vi "BeamAnalyzer.vi"() -> ()   [LabVIEW 2011]
uses:
  <vilib>/Utility/miscctls.llb/LVCursorListTypeDef.ctl
  <vilib>/gmath/NI_Gmath.lvlib
panel:
  out "Numeric system matrix":dbl[][][](array[numeric])=[[[1.0, 0.0, 0.0, 0.0], [0.0, 1.0, 0.0, 0.0], [0.0, 0.0, 1.0, 0.0], [0.0, 0.0, 0.0, 1.0]], [[1.0, 80.487805, 0.0, 0.0], [-0.03333333333333333, -1.6829268333333331, 0.0, 0.0], [0.0, 0.0, 1.0, 80.487805], [0.0, 0.0, -0.03333333333333333, -1.6829268333333331]]]
  in  "Plot system fast":bool
  out "error":i32
  in  "number of points":u32=100
  out "Y array":dbl[][][](array[numeric])=[[[0.016448811606198852, 0.029859124074476537, 0.05248408284624274, 0.07654801361501866, 0.10102784566185909, 0.12568078844527222, 0.15042175156489726, 0.17521345233159344, 0.2000370270388385, 0.22488192072640245, 0.24974177088971808, 0.27461251566370104, 0.29949144088878066, 0.3243766643064927, 0.34926683968286143, 0.37416097876713134, 0.3990583397654776, 0.42395835504829776, 0.448860582885839, 0.47376467438639763, 0.49867035033051754, 0.5235773846104799, 0.5484855921779689, 0.5733948201305636, 0.5983049410232071, 0.6232158477826785, 0.6481274497941432, 0.6730396698563271, 0.6979524417884401, 0.7228657085317128, 0.7477794206302699, 0.7726935350057659, 0.797608013961588, 0.8225228243679736, 0.847437936990825, 0.8723533259355064, 0.8972689681832823, 0.9221848432028807, 0.9471009326233549, 0.9720172199572462, 0.9969336903652497, 1.0218503304553048, 1.0467671281103703, 1.0716840723402246, 1.0966011531534607, 1.121518361446548, 1.146435688907353, 1.1713531279309763, 1.1962706715461031, 1.2211883133503711, 1.246106047453491, 1.2710238684270556, 1.2959417712601402, 1.3208597513199272, 1.3457778043167032, 1.3706959262726768, 1.395614113494133, 1.4205323625465187, 1.4454506702321086, 1.470369033569936, 1.4952874497777342, 1.5202059162556534, 1.5451244305715506, 1.5700429904476831, 1.5949615937486477, 1.619880238470433, 1.644798922730467, 1.6697176447585562, 1.6946364028886234, 1.7195551955511643, 1.7444740212663505, 1.769392878637714, 1.7943117663463615, 1.8192306831456588, 1.844149627856351, 1.8690685993620708, 1.893987596605201, 1.918906618583061, 1.9438256643443839, 1.9687447329860648, 1.9936638236501494, 2.018582935521049, 2.043502067822955, 2.0684212198174454, 2.0933403908012576, 2.1182595801042217, 2.143178787087335, 2.168098011140974, 2.1930172516832216, 2.217936508158313, 2.242855780035183, 2.267775066806107, 2.2926943679854364, 2.317613683108406, 2.342533011730029, 2.3674523534240524, 2.3923717077819844, 2.417291074412175, 2.442210452938962, 2.4671298430018562], [0.016448811606198852, 0.029859124074476537, 0.05248408284624274, 0.07654801361501866, 0.10102784566185909, 0.12568078844527222, 0.15042175156489726, 0.17521345233159344, 0.2000370270388385, 0.22488192072640245, 0.24974177088971808, 0.27461251566370104, 0.29949144088878066, 0.3243766643064927, 0.34926683968286143, 0.37416097876713134, 0.3990583397654776, 0.42395835504829776, 0.448860582885839, 0.47376467438639763, 0.49867035033051754, 0.5235773846104799, 0.5484855921779689, 0.5733948201305636, 0.5983049410232071, 0.6232158477826785, 0.6481274497941432, 0.6730396698563271, 0.6979524417884401, 0.7228657085317128, 0.7477794206302699, 0.7726935350057659, 0.797608013961588, 0.8225228243679736, 0.847437936990825, 0.8723533259355064, 0.8972689681832823, 0.9221848432028807, 0.9471009326233549, 0.9720172199572462, 0.9969336903652497, 1.0218503304553048, 1.0467671281103703, 1.0716840723402246, 1.0966011531534607, 1.121518361446548, 1.146435688907353, 1.1713531279309763, 1.1962706715461031, 1.2211883133503711, 1.246106047453491, 1.2710238684270556, 1.2959417712601402, 1.3208597513199272, 1.3457778043167032, 1.3706959262726768, 1.395614113494133, 1.4205323625465187, 1.4454506702321086, 1.470369033569936, 1.4952874497777342, 1.5202059162556534, 1.5451244305715506, 1.5700429904476831, 1.5949615937486477, 1.619880238470433, 1.644798922730467, 1.6697176447585562, 1.6946364028886234, 1.7195551955511643, 1.7444740212663505, 1.769392878637714, 1.7943117663463615, 1.8192306831456588, 1.844149627856351, 1.8690685993620708, 1.893987596605201, 1.918906618583061, 1.9438256643443839, 1.9687447329860648, 1.9936638236501494, 2.018582935521049, 2.043502067822955, 2.0684212198174454, 2.0933403908012576, 2.1182595801042217, 2.143178787087335, 2.168098011140974, 2.1930172516832216, 2.217936508158313, 2.242855780035183, 2.267775066806107, 2.2926943679854364, 2.317613683108406, 2.342533011730029, 2.3674523534240524, 2.3923717077819844, 2.417291074412175, 2.442210452938962, 2.4671298430018562]]]
  out "X":dbl[][](array[numeric])=[[0.0, 1.515, 3.03, 4.545, 6.06, 7.574999999999999, 9.09, 10.604999999999999, 12.12, 13.635, 15.149999999999999, 16.665, 18.18, 19.695, 21.209999999999997, 22.724999999999998, 24.24, 25.755, 27.27, 28.784999999999997, 30.299999999999997, 31.814999999999998, 33.33, 34.845, 36.36, 37.875, 39.39, 40.904999999999994, 42.419999999999995, 43.934999999999995, 45.449999999999996, 46.964999999999996, 48.48, 49.995, 51.51, 53.025, 54.54, 56.055, 57.56999999999999, 59.084999999999994, 60.599999999999994, 62.114999999999995, 63.629999999999995, 65.145, 66.66, 68.175, 69.69, 71.205, 72.72, 74.235, 75.75, 77.265, 78.78, 80.295, 81.80999999999999, 83.32499999999999, 84.83999999999999, 86.35499999999999, 87.86999999999999, 89.38499999999999, 90.89999999999999, 92.41499999999999, 93.92999999999999, 95.445, 96.96, 98.475, 99.99, 101.505, 103.02, 104.535, 106.05, 107.565, 109.08, 110.595, 112.11, 113.62499999999999, 115.13999999999999, 116.65499999999999, 118.16999999999999, 119.68499999999999, 121.19999999999999, 122.71499999999999, 124.22999999999999, 125.74499999999999, 127.25999999999999, 128.775, 130.29, 131.80499999999998, 133.32, 134.83499999999998, 136.35, 137.86499999999998, 139.38, 140.89499999999998, 142.41, 143.92499999999998, 145.44, 146.95499999999998, 148.47, 149.98499999999999]]
  in  "Wavelength":dbl=0.00085
  out "q out":T1(array[cluster])=[{"qx"={"Re"="((z)*((1)+(0)*(0))+(1)*((1)*(0)+(0)*((1)^2 +(0)^2)))/((1)^2 + 2*(0)*(1)*(0)+(0)^2 *((1)^2 + (0)^2))", "Im"="(-(z)*(0)*(1)+(1)*(1)*(1))/((1)^2 + 2*(0)*(1)*(0)+(0)^2 *((1)^2 +(0)^2))"}, "qy"={"Re"="((z)*((1)+(0)*(0))+(1)*((1)*(0)+(0)*((1)^2 +(0)^2)))/((1)^2 + 2*(0)*(1)*(0)+(0)^2 *((1)^2 + (0)^2))", "Im"="(-(z)*(0)*(1)+(1)*(1)*(1))/((1)^2 + 2*(0)*(1)*(0)+(0)^2 *((1)^2 +(0)^2))"}}]
  in  "q in":T2={"qx"={"Re"="0", "Im"="1"}, "qy"={"Re"="0", "Im"="1"}}
  in  "Parameters":cluster{"Name":string, "Value":string}[](array[cluster])=[{"Name"="d0", "Value"="0"}, {"Name"="z", "Value"="x"}, {"Name"="f1", "Value"="30"}, {"Name"="d1", "Value"="80.487805"}]
  out "System plot":cluster{dbl[], dbl[]}[](graph)
  in  "Plot system":bool
  in  "LensHeight":u32=20
  out "Axis vertical pos":i16=63
  in  "Horizontal initial pos":dbl
  out "Horizontal pixels":u32=898
  in  "Horizontal final point":dbl=200.0
  in  "System matrix":string[][][](array[string])=[[["1", "z", "0", "0"], ["0", "1", "0", "0"], ["0", "0", "1", "z"], ["0", "0", "0", "1"]]]
  in  "Compute System":bool
  in  "Element cluster":T3
  in  "Element array":T4(array[cluster])=[{"Element type"="Spherical lens", "Position"="80.487805", "Parameters"=[{"Name"="f1", "Value"="30"}, {"Name"="d1", "Value"="80.487805"}]}]
  in  "Stop":bool
  in  "Objects":T5(tab)
  in  "Lens type":T6(radio)
  in  "Position":string="150"
  in  "Focal length":string="100"
  in  "Add lens":bool
  out "System plot":picture
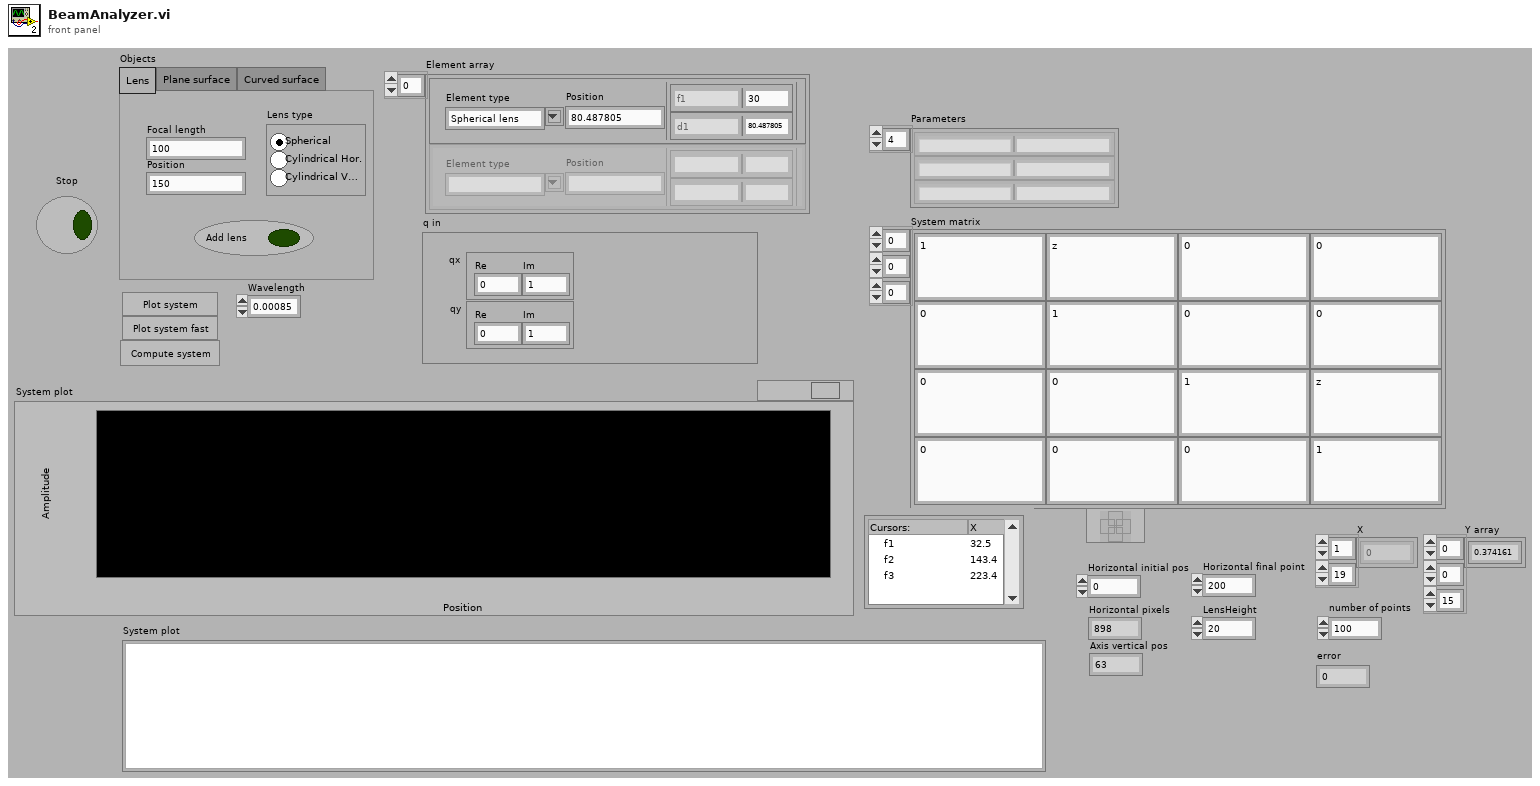
[diagram p1: front panel]
types:
  T1 = cluster{"qx":cluster{"Re":string, "Im":string}, "qy":cluster{"Re":string, "Im":string}}[]
  T2 = cluster{"qx":cluster{"Re":string, "Im":string}, "qy":cluster{"Re":string, "Im":string}}
  T3 = cluster{"Element type":string, "Position":string, "Parameters":cluster{"Name":string, "Value":string}[]}
  T4 = cluster{"Element type":string, "Position":string, "Parameters":cluster{"Name":string, "Value":string}[]}[]
  T5 = enum32{"Lens", "Plane surface", "Curved surface"}
  T6 = enum32{"Spherical", "Cylindrical Hor.", "Cylindrical Vert."}
  T7 = typedef "LVCursorListTypeDef.ctl" = cluster{"Name":string, "Color":u32, "Style":u8, "Point Style":u8, "Name Visible":bool, "Allow Drag":bool, "Cursor Mode":u32, "Plot":i32, "Index":i32, "Position":cluster{"X":dbl, "Y":dbl}, "X Scale":u32, "Y Scale":u32, "Watch Plots":i32[], "Watch All Plots":bool, "Plot Area":i32, "Label Offset":cluster{"X":dbl, "Y":dbl}}[]
  T8 = cluster{"Name":string, "Color":u32, "Style":u8, "Point Style":u8, "Name Visible":bool, "Allow Drag":bool, "Cursor Mode":u32, "Plot":i32, "Index":i32, "Position":cluster{"X":dbl, "Y":dbl}, "X Scale":u32, "Y Scale":u32, "Watch Plots":i32[], "Watch All Plots":bool, "Plot Area":i32, "Label Offset":cluster{"X":dbl, "Y":dbl}}
  T9 = typedef "LVBoundsTypeDef.ctl" = cluster{"Width":u32, "Height":u32}
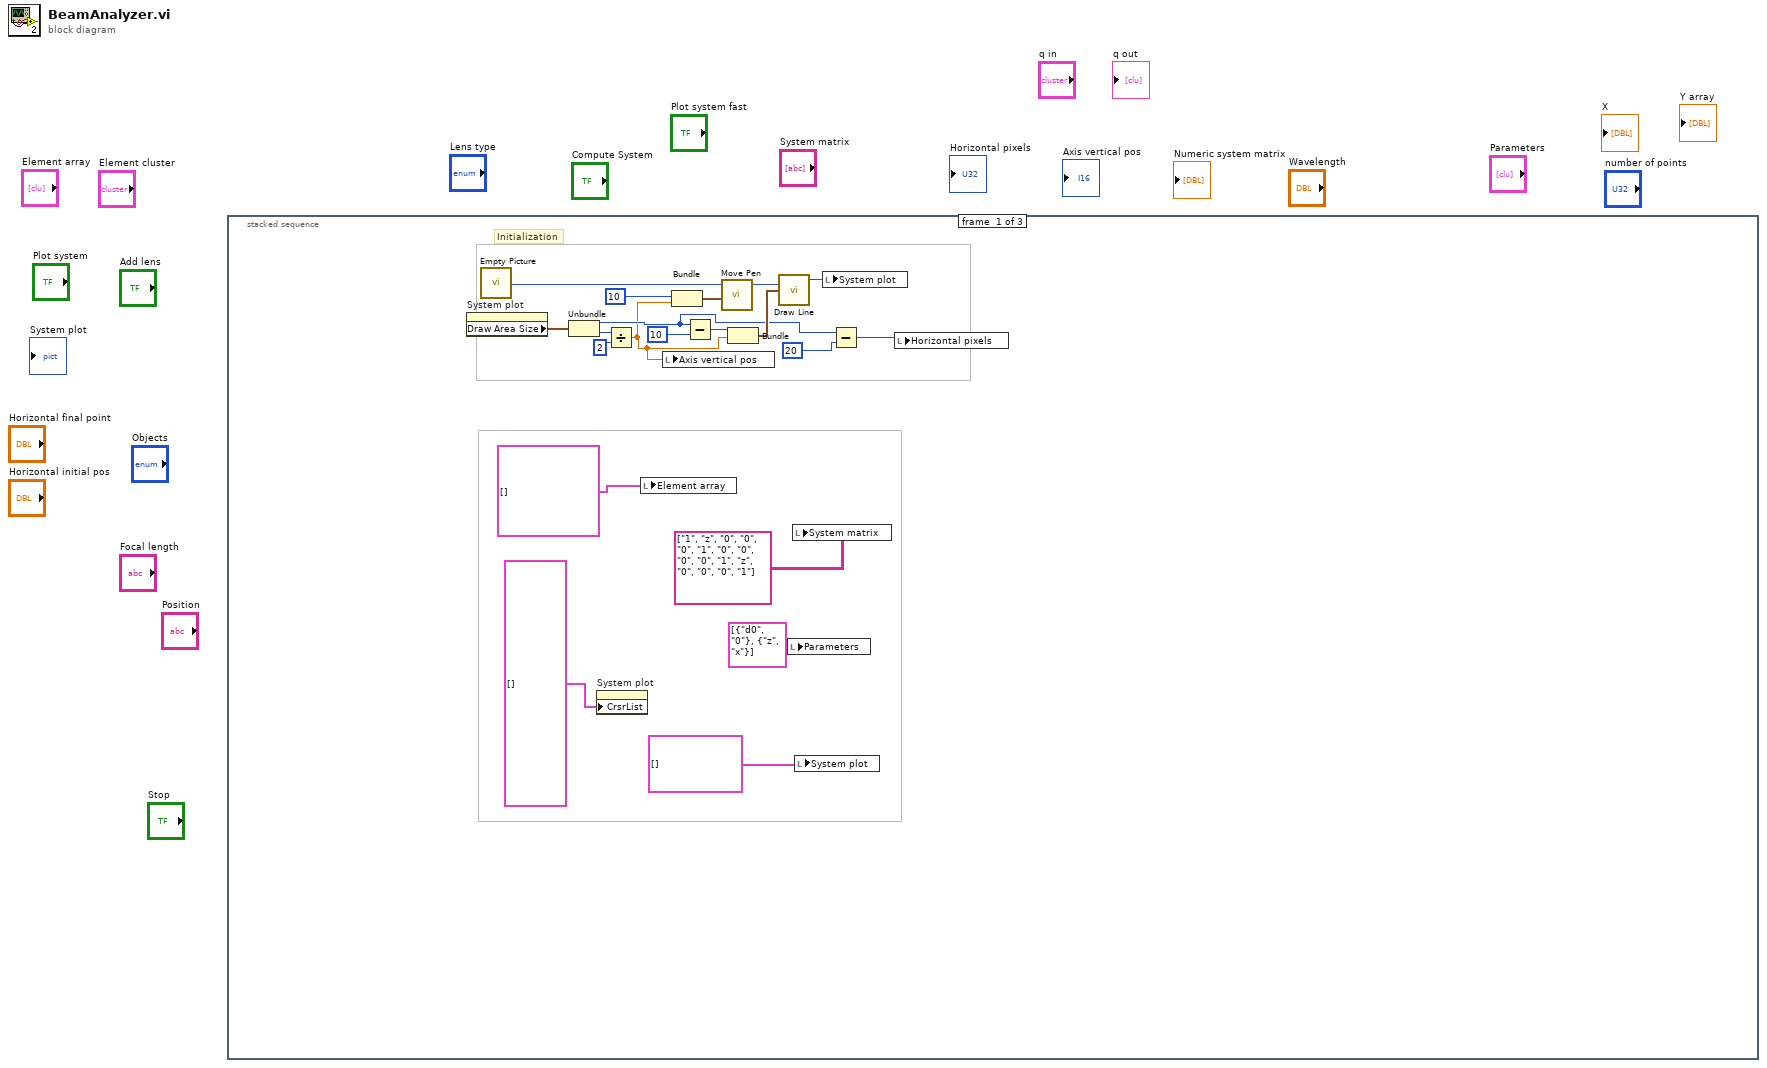
[diagram p0: block diagram]
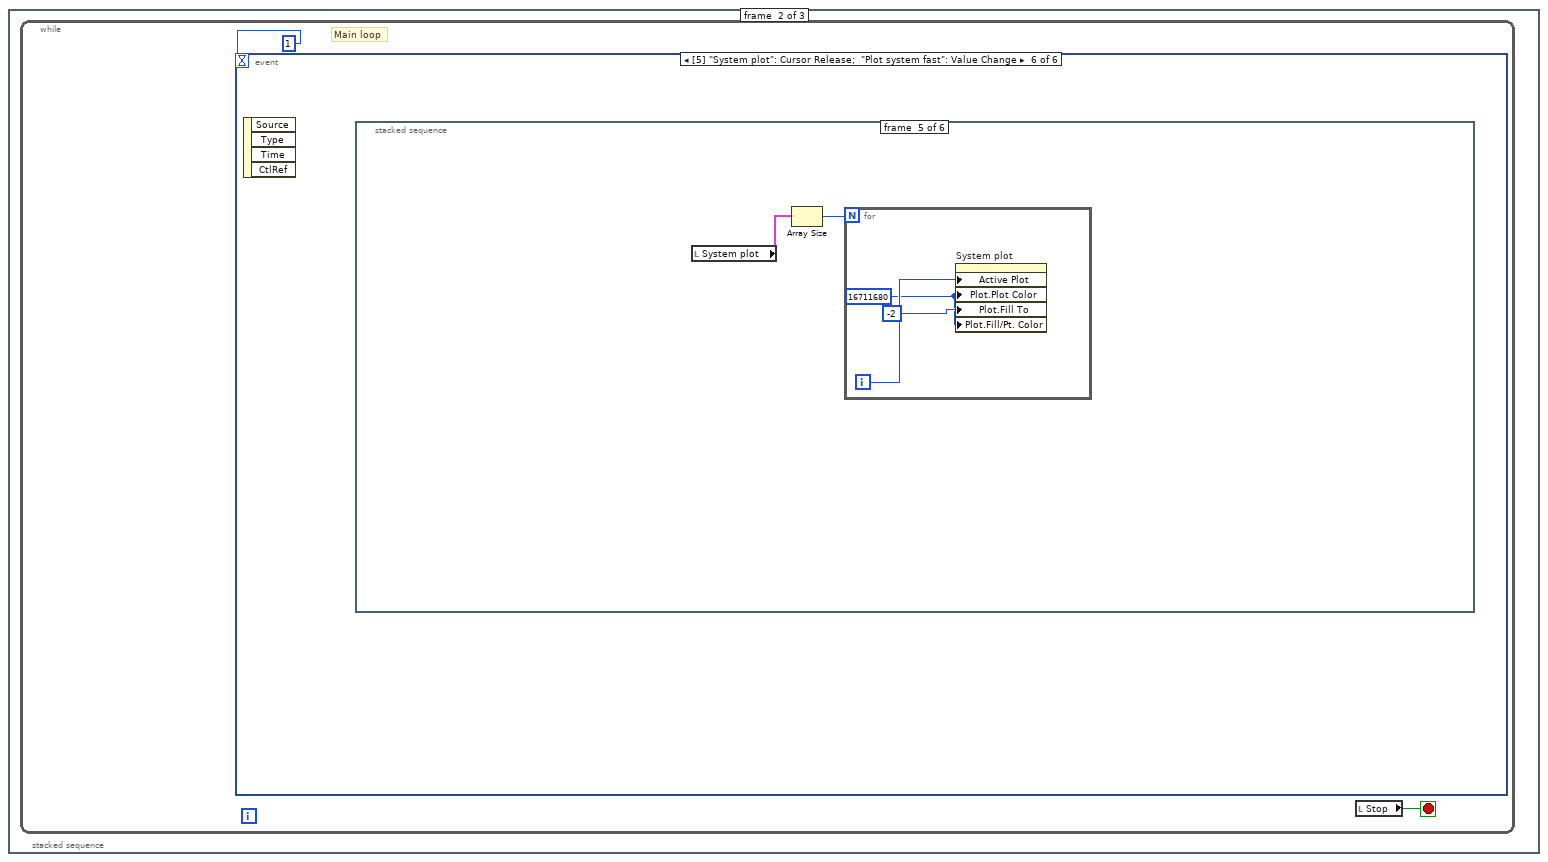
[diagram p2: hidden frame]
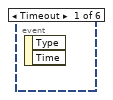
[diagram p3: hidden frame]
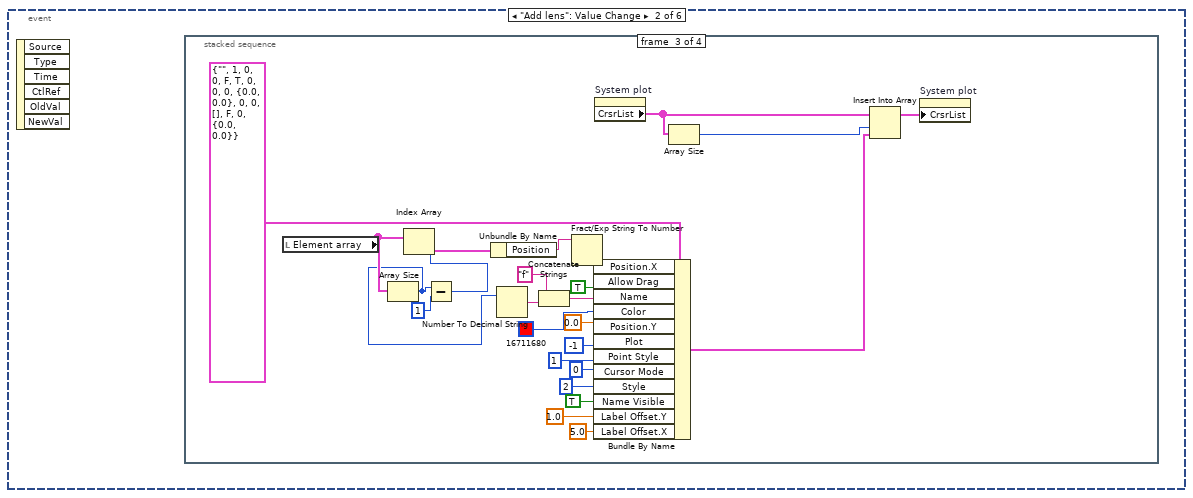
[diagram p4: hidden frame]
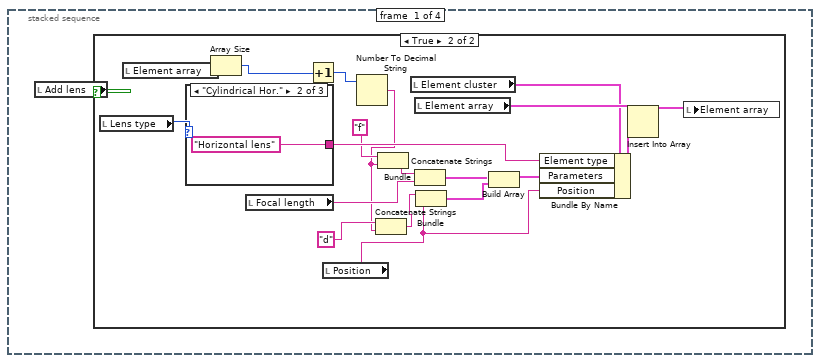
[diagram p5: hidden frame]
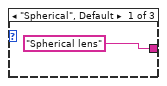
[diagram p7: hidden frame]
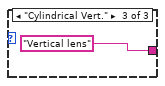
[diagram p8: hidden frame]
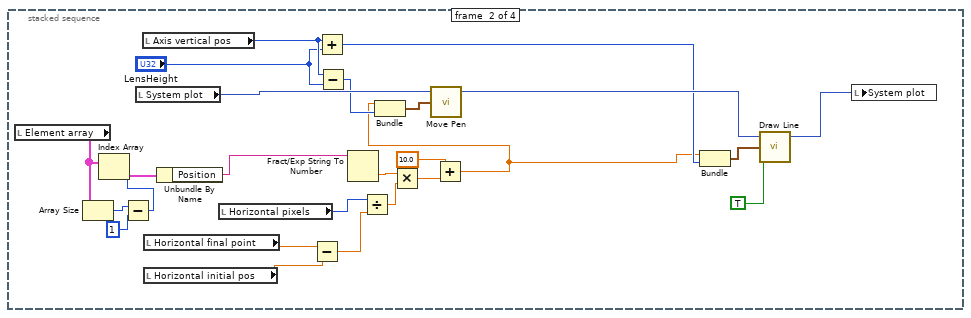
[diagram p9: hidden frame]
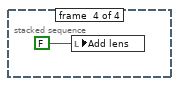
[diagram p10: hidden frame]
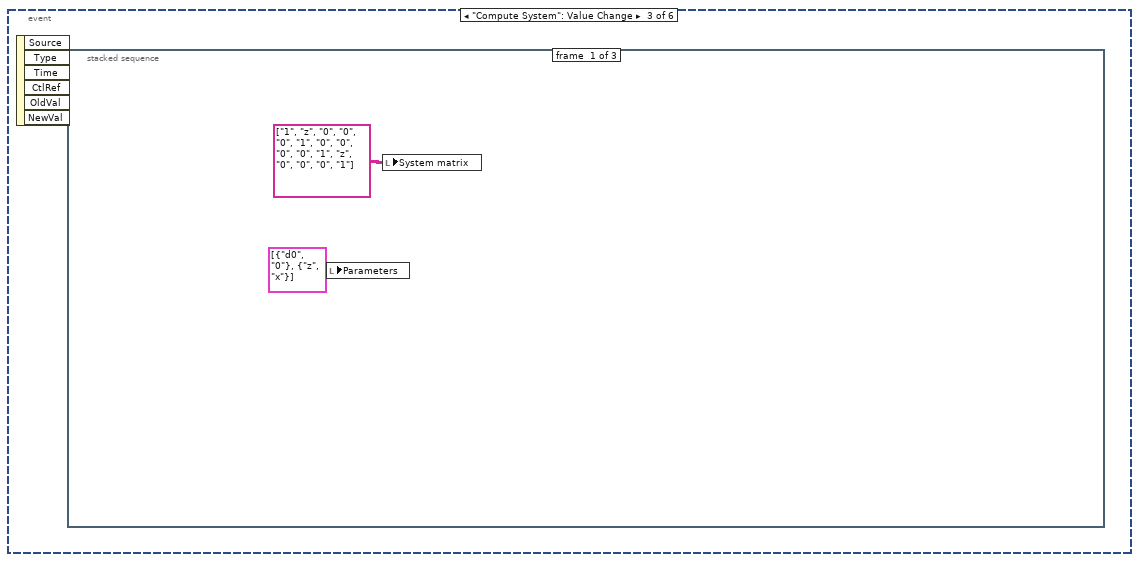
[diagram p11: hidden frame]
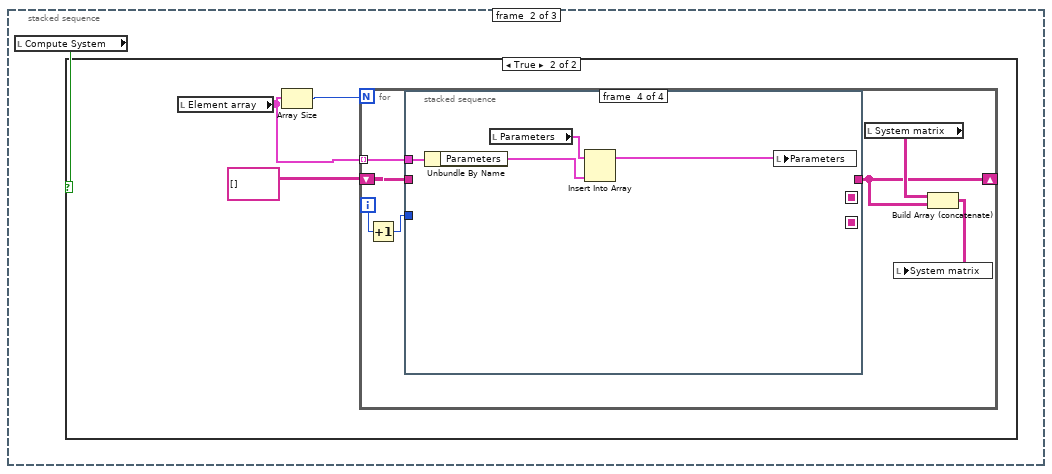
[diagram p12: hidden frame]
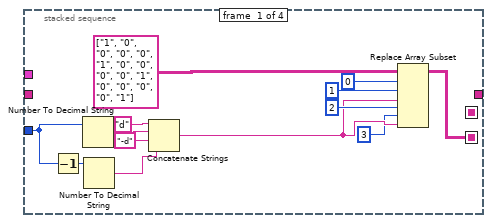
[diagram p14: hidden frame]
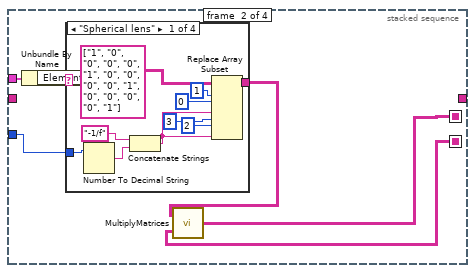
[diagram p15: hidden frame]
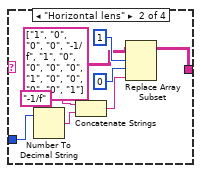
[diagram p16: hidden frame]
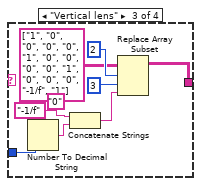
[diagram p17: hidden frame]
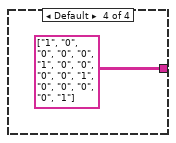
[diagram p18: hidden frame]
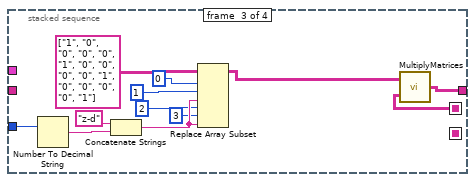
[diagram p19: hidden frame]
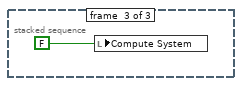
[diagram p20: hidden frame]
diagram:
  n1 = stacked-sequence {
    frame #0 {
      # "Initialization"
      n2 = property on="System plot" class="Pict"() -> ("Draw Area Size"=w17:T9)  [unwired: 2 in, 2 out]
      n3 = call "Empty Picture"() -> ("empty picture"=w18:picture)
      n4 = Unbundle(w17) -> ("Width"=w9:u32, "Height"=w16:u32)
      n5 = property on="System plot" class="XYGraph (strict)"("CrsrList"=T7 [] ("Cursor List")) -> ()  [unwired: 2 in, 2 out]
      n6 = Divide(x=w16, y=u32 2) -> (x/y=w5:dbl)
      n7 = local write "Element array"(T4 [] ("Element array")) -> ()
      n8 = local write "Axis vertical pos"(w5) -> ()
      n9 = Bundle("x"=u32 10, w5) -> (w13:cluster{"x":u32, dbl})  [unwired: 1 in]
      n10 = Subtract(x=w9, y=u32 10) -> (x-y=w6:u32)
      n11 = call <vilib>:"Move Pen.vi"("new position"=w13, "picture"=w18) -> ("new picture"=w20:picture)  [unwired: 3 in]
      n12 = Bundle(w6, w5) -> (w11:cluster{u32, dbl})  [unwired: 1 in]
      n13 = call <vilib>:"Draw Line.vi"("picture"=w20, "end point"=w11) -> ("new picture"=w19:picture)  [unwired: 7 in]
      n14 = local write "Parameters"(cluster{"Name":string, "Value":string}[] [{"Name"="d0", "Value"="0"}, {"Name"="z", "Value"="x"}] ("Parameters")) -> ()
      n15 = local write "System matrix"(string[][][] [[["1", "z", "0", "0"], ["0", "1", "0", "0"], ["0", "0", "1", "z"], ["0", "0", "0", "1"]]] ("Matrix3")) -> ()
      n16 = local write "System plot"(cluster{dbl[], dbl[]}[] []) -> ()
      n17 = local write "System plot"(w19) -> ()
      n18 = Subtract(x=w9, y=u32 20) -> (x-y=w7:u32)
      n19 = local write "Horizontal pixels"(w7) -> ()
    }
    frame #1 {
      n20 = while {
        stop <- w22 stop-if-true
        # "Main loop"
        n21 = event shown="[5] \"System plot\": Cursor Release;  \"Plot system fast\": Value Change" {
          selector: _ -> [_ _ _ _ _ _]
          dyn-events: _ -> [_ _ _ _ _ _]
          timeout: 1 ("Numeric") -> [_ _ _ _ _ _]
          event Timeout {
            n22 = event-data() -> ()  [unwired: 1 in, 2 out]
          }
          event "Add lens": Value Change {
            n23 = event-data() -> ()  [unwired: 1 in, 6 out]
            n24 = stacked-sequence {
              frame #0 {
                n25 = local read "Add lens"() -> (w23:bool)
                n26 = case shown="True" w23 {
                  frame False {
                  }
                  frame True {
                    n27 = local read "Lens type"() -> (w34:T6)
                    n28 = local read "Element array"() -> (w31:T4)
                    n29 = case shown="\"Cylindrical Hor.\"" w34 {
                      tunnel: ["Spherical lens" "Horizontal lens" "Vertical lens"] -> w35
                      frame "Spherical", Default {
                      }
                      frame "Cylindrical Hor." {
                      }
                      frame "Cylindrical Vert." {
                      }
                    }
                    n30 = Array Size(array=w31) -> (size(s)=w25:i32)
                    n31 = local read "Focal length"() -> (w37:string)
                    n32 = Increment(x=w25) -> (x+1=w24:i32)
                    n33 = local read "Position"() -> (w26:string)
                    n34 = Number To Decimal String(number=w24) -> (decimal integer string=w27:string)  [unwired: 1 in]
                    n35 = Concatenate Strings("d" ("string"), w27) -> (w29:string)
                    n36 = Concatenate Strings("f" ("string"), w27) -> (w33:string)
                    n37 = local read "Element cluster"() -> (w40:T3)
                    n38 = local read "Element array"() -> (w41:T4)
                    n39 = Bundle(w33, "Focal length"=w37) -> (w36:cluster{string, "Focal length":string})  [unwired: 1 in]
                    n40 = Bundle(w29, "Position"=w26) -> (w30:cluster{string, "Position":string})  [unwired: 1 in]
                    n41 = Build Array(w36, w30) -> (w38:cluster{string, "Position":string}[])
                    n42 = Bundle By Name(cluster=w40, "Element type"=w35, "Parameters"=w38, "Position"=w26) -> (w42:T3)
                    n43 = Insert Into Array(array=w41, new element=w42) -> (w39:T4)  [unwired: 1 in]
                    n44 = local write "Element array"(w39) -> ()
                  }
                }
              }
              frame #1 {
                n45 = local read "Element array"() -> (w50:T4)
                n46 = Array Size(array=w50) -> (size(s)=w49:i32)
                n47 = Subtract(x=w49, y=1) -> (x-y=w47:i32)
                n48 = Index Array(array=w50, index=w47) -> (element=w46:T3)
                n49 = local read "System plot"() -> (w59:picture)
                n50 = local read "Axis vertical pos"() -> (w61:i16)
                n51 = local read "Horizontal final point"() -> (w69:dbl)
                n52 = local read "Horizontal initial pos"() -> (w68:dbl)
                n53 = Unbundle By Name(w46) -> ("Position"=w51:string)
                n54 = local read "Horizontal pixels"() -> (w66:u32)
                n55 = Subtract(x=w69, y=w68) -> (x-y=w67:dbl)
                n56 = Add(x=w61, y="LensHeight") -> (x+y=w55:u32)
                n57 = Subtract(x=w61, y="LensHeight") -> (x-y=w56:u32)
                n58 = Fract/Exp String To Number(string=w51) -> (number=w52:dbl)  [unwired: 3 in, 1 out]
                n59 = Divide(x=w66, y=w67) -> (x/y=w65:dbl)
                n60 = Multiply(x=w52, y=w65) -> (x*y=w63:dbl)
                n61 = Add(x=10.0, y=w63) -> (x+y=w53:dbl)
                n62 = Bundle(w53, w56) -> (w57:cluster{dbl, u32})  [unwired: 1 in]
                n63 = call <vilib>:"Move Pen.vi"("new position"=w57, "picture"=w59) -> ("new picture"=w58:picture)  [unwired: 3 in]
                n64 = Bundle(w53, w55) -> (w54:cluster{dbl, u32})  [unwired: 1 in]
                n65 = call <vilib>:"Draw Line.vi"("picture"=w58, "end point"=w54, "absolute coordinates?(T)"=TRUE ("fill?(F)")) -> ("new picture"=w62:picture)  [unwired: 6 in]
                n66 = local write "System plot"(w62) -> ()
              }
              frame #2 {
                n67 = local read "Element array"() -> (w85:T4)
                n68 = Array Size(array=w85) -> (size(s)=w83:i32)
                n69 = Subtract(x=w83, y=1) -> (x-y=w88:i32)
                n70 = Index Array(array=w85, index=w88) -> (element=w87:T3)
                n71 = Unbundle By Name(w87) -> ("Position"=w86:string)
                n72 = Number To Decimal String(number=w83) -> (decimal integer string=w77:string)  [unwired: 1 in]
                n73 = Concatenate Strings("f" ("string"), w77) -> (w75:string)
                n74 = Fract/Exp String To Number(string=w86) -> (number=w94:dbl)  [unwired: 3 in, 1 out]
                n75 = Bundle By Name(cluster=T8 {"Name"="", "Color"=1, "Style"=0, "Point Style"=0, "Name Visible"=FALSE, "Allow Drag"=TRUE, "Cursor Mode"=0, "Plot"=0, "Index"=0, "Position"={"X"=0.0, "Y"=0.0}, "X Scale"=0, "Y Scale"=0, "Watch Plots"=[], "Watch All Plots"=FALSE, "Plot Area"=0, "Label Offset"={"X"=0.0, "Y"=0.0}} ("new element/subarray"), "Position.X"=w94, "Allow Drag"=TRUE, "Name"=w75, "Color"=u32 16711680, "Position.Y"=0.0, "Plot"=-1, "Point Style"=u8 1, "Cursor Mode"=u32 0, "Style"=u8 2, "Name Visible"=TRUE, "Label Offset.Y"=1.0, "Label Offset.X"=5.0) -> (w93:T8)
                n76 = property on="System plot" class="XYGraph (strict)"() -> ("CrsrList"=w91:T7)  [unwired: 2 in, 2 out]
                n77 = Array Size(array=w91) -> (size(s)=w92:i32)
                n78 = Insert Into Array(array=w91, index=w92, new element=w93) -> (w90:T7)
                n79 = property on="System plot" class="XYGraph (strict)"("CrsrList"=w90) -> ()  [unwired: 2 in, 2 out]
              }
              frame #3 {
                n80 = local write "Add lens"(FALSE ("Add element")) -> ()
              }
            }
          }
          event "Compute System": Value Change {
            n81 = event-data() -> ()  [unwired: 1 in, 6 out]
            n82 = stacked-sequence {
              frame #0 {
                n83 = local write "Parameters"(cluster{"Name":string, "Value":string}[] [{"Name"="d0", "Value"="0"}, {"Name"="z", "Value"="x"}] ("Parameters")) -> ()
                n84 = local write "System matrix"(string[][][] [[["1", "z", "0", "0"], ["0", "1", "0", "0"], ["0", "0", "1", "z"], ["0", "0", "0", "1"]]] ("Matrix3")) -> ()
              }
              frame #1 {
                n85 = local read "Compute System"() -> (w99:bool)
                n86 = case shown="True" w99 {
                  frame False {
                  }
                  frame True {
                    n87 = local read "Element array"() -> (w102:T4)
                    n88 = Array Size(array=w102) -> (size(s)=w101:i32)
                    n89 = for {
                      N: w101 -> [_]
                      tunnel: w102 -> [w109] mode=indexing
                      shift-right: [w105] -> _
                      shift-left: string[][] [] ("Matrix3") -> [w108]
                      i -> [w104]
                      n90 = Increment(x=w104) -> (x+1=w103:i32)
                      n91 = stacked-sequence {
                        seq-local: [w116 _ _ _] -> [_ w125 _ _]
                        seq-local: [_ w124 _ _] -> [_ _ w159 _]
                        tunnel: w109 -> [_ w128 _ w171]
                        tunnel: w108 -> [_ _ _ _]
                        tunnel: [_ _ w158 _] -> w105
                        tunnel: w103 -> [w111 w123 w157 _]
                        frame #0 {
                          n92 = Decrement(x=w111) -> (x-1=w112:i32)
                          n93 = Number To Decimal String(number=w111) -> (decimal integer string=w117:string)  [unwired: 1 in]
                          n94 = Number To Decimal String(number=w112) -> (decimal integer string=w114:string)  [unwired: 1 in]
                          n95 = Concatenate Strings("d" ("string"), w117, "-d" ("string"), w114) -> (w113:string)
                          n96 = Replace Array Subset(array=string[][] [["1", "0", "0", "0"], ["0", "1", "0", "0"], ["0", "0", "1", "0"], ["0", "0", "0", "1"]], new element #1=w113, index (row) #1=0 ("index (row)"), index (col) #1=1 ("disabled index (col)"), new element #2=w113, index (row) #2=2 ("index (row)"), index (col) #2=3 ("disabled index (col)")) -> (w116:string[][])
                        }
                        frame #1 {
                          n97 = Unbundle By Name(w128) -> ("Element type"=w127:string)
                          n98 = case shown="\"Spherical lens\"" w127 {
                            tunnel: [w129 w140 w148 string[][] [["1", "0", "0", "0"], ["0", "1", "0", "0"], ["0", "0", "1", "0"], ["0", "0", "0", "1"]]] -> w126
                            tunnel: w123 -> [w132 w141 w147 _]
                            frame "Spherical lens" {
                              n99 = Number To Decimal String(number=w132) -> (decimal integer string=w130:string)  [unwired: 1 in]
                              n100 = Concatenate Strings("-1/f" ("string"), w130) -> (w133:string)
                              n101 = Replace Array Subset(array=string[][] [["1", "0", "0", "0"], ["0", "1", "0", "0"], ["0", "0", "1", "0"], ["0", "0", "0", "1"]], new element #1=w133, index (row) #1=1 ("index (row)"), index (col) #1=0 ("disabled index (col)"), new element #2=w133, index (row) #2=3 ("index (row)"), index (col) #2=2 ("disabled index (col)")) -> (w129:string[][])
                            }
                            frame "Horizontal lens" {
                              n102 = Number To Decimal String(number=w141) -> (decimal integer string=w144:string)  [unwired: 1 in]
                              n103 = Concatenate Strings("-1/f" ("string"), w144) -> (w143:string)
                              n104 = Replace Array Subset(array=string[][] [["1", "0", "0", "0"], ["-1/f", "1", "0", "0"], ["0", "0", "1", "0"], ["0", "0", "0", "1"]], new element=w143, index (row)=1, index (col)=0 ("disabled index (col)")) -> (w140:string[][])
                            }
                            frame "Vertical lens" {
                              (unwired) "0"
                              n105 = Number To Decimal String(number=w147) -> (decimal integer string=w152:string)  [unwired: 1 in]
                              n106 = Concatenate Strings("-1/f" ("string"), w152) -> (w151:string)
                              n107 = Replace Array Subset(array=string[][] [["1", "0", "0", "0"], ["0", "1", "0", "0"], ["0", "0", "1", "0"], ["0", "0", "-1/f", "1"]], new element=w151, index (row)=2, index (col)=3 ("disabled index (col)")) -> (w148:string[][])
                            }
                            frame Default {
                            }
                          }
                          n108 = call "MultiplyMatrices.vi"("Matrix2"=w125, "Matrix1"=w126) -> ("Matrix3"=w124:string[][])
                        }
                        frame #2 {
                          n109 = Number To Decimal String(number=w157) -> (decimal integer string=w165:string)  [unwired: 1 in]
                          n110 = Concatenate Strings("z-d" ("string"), w165) -> (w166:string)
                          n111 = Replace Array Subset(array=string[][] [["1", "0", "0", "0"], ["0", "1", "0", "0"], ["0", "0", "1", "0"], ["0", "0", "0", "1"]], new element #1=w166, index (row) #1=0 ("index (row)"), index (col) #1=1 ("disabled index (col)"), new element #2=w166, index (row) #2=2 ("index (row)"), index (col) #2=3 ("disabled index (col)")) -> (w167:string[][])
                          n112 = call "MultiplyMatrices.vi"("Matrix2"=w159, "Matrix1"=w167) -> ("Matrix3"=w158:string[][])
                        }
                        frame #3 {
                          n113 = Unbundle By Name(w171) -> ("Parameters"=w168:cluster{"Name":string, "Value":string}[])
                          n114 = local read "Parameters"() -> (w170:cluster{"Name":string, "Value":string}[])
                          n115 = Insert Into Array(array=w170, new element=w168) -> (w169:cluster{"Name":string, "Value":string}[])  [unwired: 1 in]
                          n116 = local write "Parameters"(w169) -> ()
                        }
                      }
                      n117 = local read "System matrix"() -> (w107:string[][][])
                      n118 = Build Array (concatenate)(w107, w105) -> (w106:string[][][])
                      n119 = local write "System matrix"(w106) -> ()
                    }
                  }
                }
              }
              frame #2 {
                n120 = local write "Compute System"(FALSE ("Compute System")) -> ()
              }
            }
          }
          event "Plot system": Value Change {
            n121 = event-data() -> ()  [unwired: 1 in, 6 out]
            n122 = local read "Plot system"() -> (w173:bool)
            n123 = case shown="True" w173 {
              frame False {
              }
              frame True {
                n124 = local read "System matrix"() -> (w174:string[][][])
                n125 = Array Size(array=w174) -> (size(s)=w177:i32[])
                n126 = Index Array(array=w177, index=0) -> (element=w175:i32)
                n127 = stacked-sequence {
                  tunnel: w175 -> [w179 w197 _]
                  tunnel: w174 -> [w178 _ _]
                  frame #0 {
                    n128 = local read "q in"() -> (w181:T2)
                    n129 = for {
                      N: w179 -> [_]
                      tunnel: w178 -> [w184] mode=indexing
                      tunnel: w181 -> [w183]
                      tunnel: [w182] -> w180 mode=indexing
                      n130 = call "PropagateBeam.vi"("q in"=w183, "Matrix"=w184) -> ("q out"=w182:T2)
                    }
                    n131 = local write "q out"(w180) -> ()
                  }
                  frame #1 {
                    n132 = local read "Element array"() -> (w193:T4)
                    n133 = local read "Parameters"() -> (w190:cluster{"Name":string, "Value":string}[])
                    n134 = local read "q out"() -> (w196:T1)
                    n135 = Array Size(array=w190) -> (size(s)=w195:i32)
                    n136 = local read "Horizontal initial pos"() -> (w188:dbl)
                    n137 = local read "Horizontal final point"() -> (w189:dbl)
                    n138 = Array Size(array=w193) -> (size(s)=w192:i32)
                    n139 = for {
                      N: w195 -> [_]
                      tunnel: w190 -> [w205] mode=indexing
                      tunnel: [w201] -> w194 mode=indexing
                      n140 = Unbundle(w205) -> ("Name"=w203:string, "Value"=w204:string)
                      n141 = Fract/Exp String To Number(string=w204) -> (number=w202:dbl)  [unwired: 3 in, 1 out]
                      n142 = Bundle("Name"=w203, w202) -> (w201:cluster{"Name":string, dbl})  [unwired: 1 in]
                    }
                    n143 = for {
                      N: w192 -> [_]
                      tunnel: w193 -> [w200] mode=indexing
                      tunnel: [w198] -> w191 mode=indexing
                      n144 = Unbundle By Name(w200) -> ("Position"=w199:string)
                      n145 = Fract/Exp String To Number(string=w199) -> (number=w198:dbl)  [unwired: 3 in, 1 out]
                    }
                    n146 = Build Array (concatenate)(w188, w191, w189) -> (w185:dbl[])
                    n147 = for {
                      N: w197 -> [_]
                      tunnel: w196 -> [w224] mode=indexing
                      tunnel: w194 -> [w222]
                      tunnel: w185 -> [w221]
                      tunnel: [w216] -> w186 mode=indexing
                      tunnel: [w215] -> w187 mode=indexing
                      tunnel: w190 -> [w217]
                      tunnel: [w212] -> _ mode=indexing
                      i -> [w220]
                      w218 = 2
                      n148 = Cluster To Array(cluster=w224) -> (array=w223:cluster{"Re":string, "Im":string}[])
                      n149 = Increment(x=w220) -> (x+1=w219:i32)
                      n150 = Index Array(array=w221, index #1=w220, index #2=w219) -> (element #1=w210:dbl, element #2=w211:dbl)
                      n151 = local read "number of points"() -> (w208:u32)
                      n152 = Subtract(x=w211, y=w210) -> (x-y=w209:dbl)
                      n153 = Divide(x=w209, y=w208) -> (x/y=w207:dbl)
                      n154 = Add(x=w207, y=w211) -> (x+y=w206:dbl)
                      n155 = for {
                        N: w218 -> [_]
                        tunnel: w223 -> [w246] mode=indexing
                        tunnel: w222 -> [w244]
                        tunnel: w210 -> [w225]
                        tunnel: w206 -> [w243]
                        tunnel: [w226] -> w216
                        tunnel: w218 -> [w242]
                        tunnel: [w231] -> w215 mode=indexing
                        tunnel: w217 -> [w230]
                        n156 = Cluster To Array(cluster=w246) -> (array=w245:string[])
                        n157 = for {
                          N: w242 -> [_]
                          tunnel: w245 -> [w250] mode=indexing
                          tunnel: w244 -> [w249]
                          tunnel: w225 -> [w256]
                          tunnel: w243 -> [w254]
                          tunnel: [w255] -> w226
                          tunnel: [w253] -> w241 mode=indexing
                          tunnel: w230 -> [w248]
                          n158 = local read "number of points"() -> (w252:u32)
                          n159 = call <vilib>:"Substitute Variables.vi"("Substitution Rules"=w248, "original formula"=w250) -> ("formula after substitution"=w247:string)  [unwired: 1 in, 1 out]
                          n160 = call <vilib>:"Eval y=f(a,x).vi"("number of points"=w252, "formula"=w247, "Parameters"=w249, "end"=w254, "start"=w256) -> ("error"=→"error":i32, "Y"=w253:dbl[], "X"=w255:dbl[])  [unwired: 1 out]
                        }
                        n161 = local read "Wavelength"() -> (w237:dbl)
                        n162 = Index Array(array=w241, index (row) #1=0 ("disabled index (col)"), index (row) #2=1 ("disabled index (col)")) -> (element #1=w229:dbl[], element #2=w234:dbl[])  [unwired: 2 in]
                        n163 = Square(x=w229) -> (x^2=w240:dbl[])
                        n164 = Square(x=w234) -> (x^2=w239:dbl[])
                        n165 = Add(x=w240, y=w239) -> (x+y=w238:dbl[])
                        n166 = Multiply(x=w234, y=3.141592653589793) -> (x*y=w233:dbl[])
                        n167 = Multiply(x=w238, y=w237) -> (x*y=w236:dbl[])
                        n168 = Divide(x=w236, y=w233) -> (x/y=w232:dbl[])
                        n169 = Square Root(x=w232) -> (sqrt(x)=w231:dbl[])
                      }
                      n170 = Index Array(array=w215, index (row)=0) -> (element=w213:dbl[])  [unwired: 1 in]
                      n171 = Bundle("X"=w216, w213) -> (w212:cluster{"X":dbl[], dbl[]})  [unwired: 1 in]
                    }
                    n172 = local write "Y array"(w187) -> ()
                    n173 = local write "X"(w186) -> ()
                  }
                  frame #2 {
                    n174 = local write "Plot system"(FALSE ("Plot system")) -> ()
                  }
                }
              }
            }
          }
          event "System plot": Cursor Move {
            n175 = event-data() -> ("CursIdx"=w259:i32, "CursLoc"=w279:cluster{"X":dbl, "Y":dbl})  [unwired: 1 in, 7 out]
            n176 = Unbundle(w279) -> ("X"=w274:dbl)  [unwired: 1 out]
            n177 = local read "Element array"() -> (w278:T4)
            n178 = local read "Parameters"() -> (w262:cluster{"Name":string, "Value":string}[])
            n179 = Increment(x=w259) -> (x+1=w258:i32)
            n180 = Number To Decimal String(number=w258) -> (decimal integer string=w267:string)  [unwired: 1 in]
            n181 = Number To Fractional String(number=w274) -> (F-format string=w264:string)  [unwired: 3 in]
            n182 = Array Size(array=w262) -> (size(s)=w261:i32)
            n183 = Concatenate Strings("d" ("string"), w267) -> (w266:string)
            n184 = Index Array(array=w278, index=w259) -> (element=w276:T3)
            n185 = while {
              tunnel: w262 -> [w295] mode=indexing
              tunnel: w266 -> [w294]
              tunnel: [w293] -> w265
              tunnel: [w292] -> _
              tunnel: [w290] -> w263
              tunnel: w261 -> [w289]
              tunnel: [w287] -> w260
              i -> [w290]
              stop <- w288 stop-if-true
              n186 = Unbundle By Name(w295) -> ("Name"=w293:string, "Value"=w292:string)
              n187 = Greater Or Equal?(x=w290, y=w289) -> (x >= y?=w287:bool)
              n188 = Equal?(x=w293, y=w294) -> (x = y?=w291:bool)
              n189 = Or(x=w291, y=w287) -> (x .or. y?=w288:bool)
            }
            n190 = Unbundle(w276) -> ("Element type"=w280:string, "Parameters"=w272:cluster{"Name":string, "Value":string}[])  [unwired: 1 out]
            n191 = while {
              tunnel: w272 -> [w300] mode=indexing
              tunnel: [w298] -> w273
              tunnel: [w297] -> w271
              tunnel: w266 -> [w296]
              i -> [w298]
              stop <- w299 stop-if-true
              n192 = Unbundle By Name(w300) -> ("Name"=w297:string)  [unwired: 1 out]
              n193 = Equal?(x=w297, y=w296) -> (x = y?=w299:bool)
            }
            n194 = Bundle("Name"=w271, w264) -> (w270:cluster{"Name":string, string})  [unwired: 1 in]
            n195 = Replace Array Subset(array=w272, new element=w270, index=w273) -> (w269:cluster{"Name":string, "Value":string}[])
            n196 = Bundle(cluster=w276, "Element type"=w280, "Position"=w264, "Parameters"=w269) -> (w277:T3)
            n197 = Replace Array Subset(array=w278, new element=w277, index=w259) -> (w275:T4)
            n198 = local write "Element array"(w275) -> ()
            n199 = case shown="False" w260 {
              tunnel: w265 -> [w286 _]
              tunnel: w264 -> [w285 _]
              tunnel: w263 -> [w283 _]
              tunnel: w262 -> [w281 _]
              frame False {
                n200 = Bundle("Name"=w286, w285) -> (w284:cluster{"Name":string, string})  [unwired: 1 in]
                n201 = Replace Array Subset(array=w281, new element=w284, index=w283) -> (w282:cluster{"Name":string, "Value":string}[])
                n202 = local write "Parameters"(w282) -> ()
              }
              frame True {
              }
            }
          }
          event "System plot": Cursor Release; "Plot system fast": Value Change {
            n203 = event-data() -> ()  [unwired: 1 in, 4 out]
            n204 = stacked-sequence {
              frame #0 {
                n205 = local write "Parameters"(cluster{"Name":string, "Value":string}[] [{"Name"="d0", "Value"="0"}, {"Name"="z", "Value"="x"}] ("Parameters")) -> ()
                n206 = property on="System plot" class="XYGraph (strict)"("Active Plot"=u32 0, "Value"=cluster{dbl[], dbl[]}[] []) -> ()  [unwired: 2 in, 2 out]
              }
              frame #1 {
                n207 = local read "Element array"() -> (w305:T4)
                n208 = Array Size(array=w305) -> (size(s)=w304:i32)
                n209 = for {
                  N: w304 -> [_]
                  tunnel: w305 -> [w310] mode=indexing
                  tunnel: [w307] -> w306 mode=indexing
                  i -> [w309]
                  n210 = Increment(x=w309) -> (x+1=w308:i32)
                  n211 = stacked-sequence {
                    seq-local: [w317 _ _] -> [_ w329 _]
                    seq-local: [_ w328 _] -> [_ _ w362]
                    tunnel: w310 -> [_ w332 _]
                    tunnel: w308 -> [w312 w327 _]
                    tunnel: [_ _ w361] -> w307
                    frame #0 {
                      n212 = Decrement(x=w312) -> (x-1=w313:i32)
                      n213 = Number To Decimal String(number=w312) -> (decimal integer string=w318:string)  [unwired: 1 in]
                      n214 = Number To Decimal String(number=w313) -> (decimal integer string=w315:string)  [unwired: 1 in]
                      n215 = Concatenate Strings("d" ("string"), w318, "-d" ("string"), w315) -> (w314:string)
                      n216 = Replace Array Subset(array=string[][] [["1", "0", "0", "0"], ["0", "1", "0", "0"], ["0", "0", "1", "0"], ["0", "0", "0", "1"]], new element #1=w314, index (row) #1=0 ("index (row)"), index (col) #1=1 ("disabled index (col)"), new element #2=w314, index (row) #2=2 ("index (row)"), index (col) #2=3 ("disabled index (col)")) -> (w317:string[][])
                    }
                    frame #1 {
                      n217 = local read "Parameters"() -> (w324:cluster{"Name":string, "Value":string}[])
                      n218 = Unbundle By Name(w332) -> ("Element type"=w331:string, "Parameters"=w326:cluster{"Name":string, "Value":string}[])
                      n219 = Insert Into Array(array=w324, new element=w326) -> (w325:cluster{"Name":string, "Value":string}[])  [unwired: 1 in]
                      n220 = local write "Parameters"(w325) -> ()
                      n221 = case shown="\"Spherical lens\"" w331 {
                        tunnel: [w333 w344 w352 string[][] [["1", "0", "0", "0"], ["0", "1", "0", "0"], ["0", "0", "1", "0"], ["0", "0", "0", "1"]]] -> w330
                        tunnel: w327 -> [w336 w345 w351 _]
                        frame "Spherical lens" {
                          n222 = Number To Decimal String(number=w336) -> (decimal integer string=w334:string)  [unwired: 1 in]
                          n223 = Concatenate Strings("-1/f" ("string"), w334) -> (w337:string)
                          n224 = Replace Array Subset(array=string[][] [["1", "0", "0", "0"], ["0", "1", "0", "0"], ["0", "0", "1", "0"], ["0", "0", "0", "1"]], new element #1=w337, index (row) #1=1 ("index (row)"), index (col) #1=0 ("disabled index (col)"), new element #2=w337, index (row) #2=3 ("index (row)"), index (col) #2=2 ("disabled index (col)")) -> (w333:string[][])
                        }
                        frame "Horizontal lens" {
                          n225 = Number To Decimal String(number=w345) -> (decimal integer string=w348:string)  [unwired: 1 in]
                          n226 = Concatenate Strings("-1/f" ("string"), w348) -> (w347:string)
                          n227 = Replace Array Subset(array=string[][] [["1", "0", "0", "0"], ["-1/f", "1", "0", "0"], ["0", "0", "1", "0"], ["0", "0", "0", "1"]], new element=w347, index (row)=1, index (col)=0 ("disabled index (col)")) -> (w344:string[][])
                        }
                        frame "Vertical lens" {
                          (unwired) "0"
                          n228 = Number To Decimal String(number=w351) -> (decimal integer string=w356:string)  [unwired: 1 in]
                          n229 = Concatenate Strings("-1/f" ("string"), w356) -> (w355:string)
                          n230 = Replace Array Subset(array=string[][] [["1", "0", "0", "0"], ["0", "1", "0", "0"], ["0", "0", "1", "0"], ["0", "0", "-1/f", "1"]], new element=w355, index (row)=2, index (col)=3 ("disabled index (col)")) -> (w352:string[][])
                        }
                        frame Default {
                        }
                      }
                      n231 = call "MultiplyMatrices.vi"("Matrix2"=w329, "Matrix1"=w330) -> ("Matrix3"=w328:string[][])
                    }
                    frame #2 {
                      w363 = 4
                      n232 = local read "Parameters"() -> (w360:cluster{"Name":string, "Value":string}[])
                      n233 = for {
                        N: w363 -> [_]
                        tunnel: w363 -> [w367]
                        tunnel: w362 -> [w366] mode=indexing
                        tunnel: w360 -> [w365]
                        tunnel: [w364] -> w361 mode=indexing
                        n234 = for {
                          N: w367 -> [_]
                          tunnel: w366 -> [w371] mode=indexing
                          tunnel: w365 -> [w370]
                          tunnel: [w368] -> w364 mode=indexing
                          n235 = call <vilib>:"Substitute Variables.vi"("Substitution Rules"=w370, "original formula"=w371) -> ("formula after substitution"=w369:string)  [unwired: 1 in, 1 out]
                          n236 = call <vilib>:"Eval Single-Variable Scalar.vi"("formula"=w369) -> ("y value"=w368:dbl)  [unwired: 2 in, 1 out]
                        }
                      }
                    }
                  }
                }
                n237 = local write "Numeric system matrix"(w306) -> ()
              }
              frame #2 {
                n238 = local read "Numeric system matrix"() -> (w372:dbl[][][])
                n239 = Build Array (concatenate)(dbl[][] [[1.0, 0.0, 0.0, 0.0], [0.0, 1.0, 0.0, 0.0], [0.0, 0.0, 1.0, 0.0], [0.0, 0.0, 0.0, 1.0]] ("element"), w372) -> (w374:dbl[][][])
                n240 = local write "Numeric system matrix"(w374) -> ()
              }
              frame #3 {
                w389 = 2
                n241 = local read "q in"() -> (w391:T2)
                n242 = Cluster To Array(cluster=w391) -> (array=w390:cluster{"Re":string, "Im":string}[])
                n243 = local read "Element array"() -> (w378:T4)
                n244 = for {
                  N: w389 -> [_]
                  tunnel: w390 -> [w437] mode=indexing
                  tunnel: [w432] -> w388 mode=indexing
                  tunnel: w389 -> [w431]
                  n245 = Cluster To Array(cluster=w437) -> (array=w436:string[])
                  n246 = for {
                    N: w431 -> [_]
                    tunnel: w436 -> [w439] mode=indexing
                    tunnel: [w438] -> w435 mode=indexing
                    n247 = call <vilib>:"Eval Formula String.vi"("formula"=w439) -> ("y value"=w438:dbl)  [unwired: 1 in, 1 out]
                  }
                  n248 = Index Array(array=w435) -> (element #1=w434:dbl, element #2=w433:dbl)  [unwired: 2 in]
                  n249 = Re/Im To Complex(1:w433, 2:w434) -> (0:w432:cdb)
                }
                n250 = local read "Horizontal final point"() -> (w380:dbl)
                n251 = Number To Engineering String(4:w380) -> (0:w379:string)  [unwired: 3 in]
                n252 = local read "Horizontal initial pos"() -> (w385:dbl)
                n253 = local read "Numeric system matrix"() -> (w382:dbl[][][])
                n254 = local read "number of points"() -> (w386:u32)
                n255 = Array To Cluster(array=w388) -> (cluster=w387:cluster{"[0]":cdb, "[1]":cdb})
                n256 = Array Size(array=w378) -> (size(s)=w383:i32)
                n257 = for {
                  N: w383 -> [_]
                  tunnel: w378 -> [w400] mode=indexing
                  tunnel: [w399] -> w381 mode=indexing
                  n258 = Unbundle By Name(w400) -> ("Position"=w399:string)
                }
                n259 = Build Array (concatenate)(w381, w379) -> (w377:string[])
                n260 = local read "Wavelength"() -> (w384:dbl)
                n261 = while {
                  tunnel: w382 -> [w421] mode=indexing
                  shift-right: [w419] -> _
                  shift-left: w387 -> [w420]
                  tunnel: w386 -> [w404]
                  tunnel: w377 -> [w406] mode=indexing
                  tunnel: w385 -> [_]
                  tunnel: w380 -> [w410]
                  shift-right: [w408] -> _
                  shift-left: w385 -> [w407]
                  tunnel: w383 -> [w416]
                  tunnel: w384 -> [w409]
                  tunnel: [w401] -> w376 mode=indexing
                  tunnel: [w402] -> _ mode=indexing
                  tunnel: [w405] -> _ mode=indexing
                  i -> [w417]
                  stop <- w413 continue-if-true
                  n262 = call "PropagateBeamNumeric.vi"("q in"=w420, "Matrix"=w421) -> ("q out"=w419:cluster{"qx":cdb, "qy":cdb})
                  n263 = Unbundle By Name(w419) -> ("qx"=w418:cdb)
                  n264 = Fract/Exp String To Number(string=w406) -> (number=w408:dbl)  [unwired: 3 in, 1 out]
                  n265 = Subtract(x=w408, y=w407) -> (x-y=w412:dbl)
                  n266 = Increment(x=w404) -> (x+1=w403:u32)
                  n267 = Divide(x=w412, y=w404) -> (x/y=w411:dbl)
                  n268 = for {
                    N: w403 -> [_]
                    tunnel: w418 -> [w427]
                    tunnel: w411 -> [w429]
                    tunnel: w407 -> [w428]
                    tunnel: w409 -> [w425]
                    tunnel: [w424] -> w402 mode=indexing
                    tunnel: [w423] -> w405 mode=indexing
                    i -> [w430]
                    n269 = Multiply(x=w429, y=w430) -> (x*y=w422:dbl)
                    n270 = Add(x=w427, y=w422) -> (x+y=w426:cdb)
                    n271 = Add(x=w422, y=w428) -> (x+y=w423:dbl)
                    n272 = call "QtoBeamDiameter.vi"("wavelength"=w425, "q"=w426) -> ("Beam diameter"=w424:dbl)
                  }
                  n273 = Less?(x=w417, y=w416) -> (x < y?=w414:bool)
                  n274 = Greater?(x=w410, y=w408) -> (0:w415:bool)
                  n275 = And(x=w415, y=w414) -> (x .and. y?=w413:bool)
                  n276 = Bundle(w405, w402) -> (w401:cluster{dbl[], dbl[]})  [unwired: 1 in]
                }
                n277 = for {
                  tunnel: w376 -> [w398] mode=indexing
                  shift-right: [w392] -> w375
                  shift-left: w376 -> [w394]
                  n278 = Unbundle(w398) -> (w396:dbl[], w397:dbl[])
                  n279 = Negate(x=w397) -> (-x=w395:dbl[])
                  n280 = Bundle(w396, w395) -> (w393:cluster{dbl[], dbl[]})  [unwired: 1 in]
                  n281 = Insert Into Array(array=w394, new element=w393) -> (w392:cluster{dbl[], dbl[]}[])  [unwired: 1 in]
                }
                "System plot" <- w375
              }
              frame #4 {
                n282 = local read "System plot"() -> (w440:cluster{dbl[], dbl[]}[])
                n283 = Array Size(array=w440) -> (size(s)=w441:i32)
                n284 = for {
                  N: w441 -> [_]
                  i -> [w444]
                  w442 = u32 16711680 ("Plot.Plot Color")
                  n285 = property on="System plot" class="XYGraph (strict)"("Active Plot"=w444, "Plot.Plot Color"=w442, "Plot.Fill To"=i16 -2, "Plot.Fill/Pt. Color"=w442) -> ()  [unwired: 2 in, 2 out]
                }
              }
              frame #5 {
                n286 = local write "Plot system fast"(FALSE ("Compute System")) -> ()
              }
            }
          }
        }
        n287 = local read "Stop"() -> (w22:bool)
      }
    }
    frame #2 {
      n288 = local write "Stop"(FALSE ("Stop")) -> ()
    }
  }
